vi "Get Tag.vi"(7 "IFDO":T4(c390), 8 "error in 2":errorcluster, 9 "byte order (0:big-endian, network order)":T1(ring), 10 "Tag ID":T2=254 items=["NewSubfileType"=254, "ImageWidth"=256, "ImageLength"=257, "BitsPerSample"=258, "Compression"=259, "PhotometricInterpretation"=262, "StripOffsets"=273, "SamplesPerPixel"=277, "RowsPerStrip"=278, "StripByteCounts"=279, "XResolution"=282, "YResolution"=283, "ResolutionUnit"=296, "ColorMap"=320, "PlanarrConfiguration"=284, "YCbCrCoefficients"=529, "YCbCrSubSampling"=530, "YCbCrPositioning"=531, "ReferenceBlackWhite"=532, "BadFaxLines"=326, "CleanFaxData"=327, "ConsecutiveBadFaxLines"=328], 11 "File Refnum":refnum<file>) -> (0 "error out":errorcluster, 1 "Tag found?":bool, 2 "Data":variant, 3 "refnum out":refnum<file>)   [LabVIEW 2020, in "LV Tiff.lvlib"]
uses:
  LV Tiff.lvlib
  Tiff Data Type.ctl
  Tiff Tags.ctl
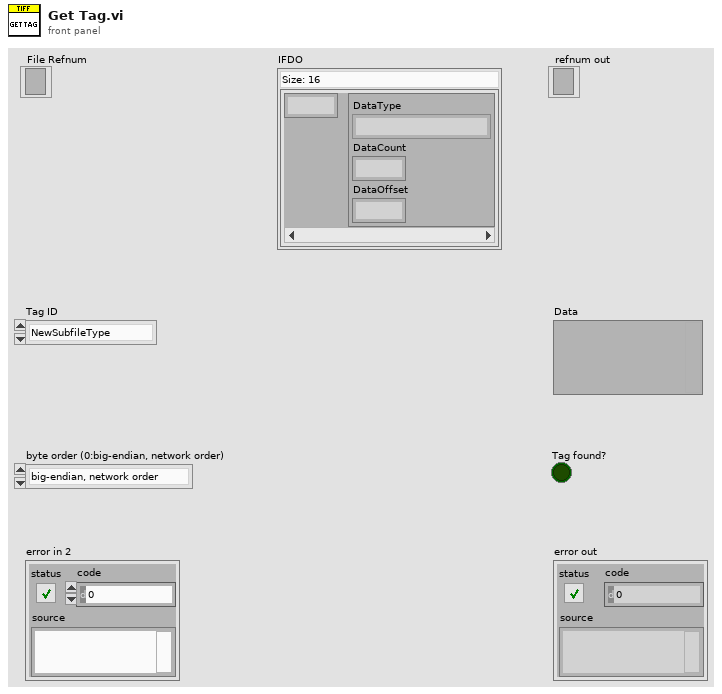
[diagram p1: front panel]
types:
  T1 = enum16{"big-endian, network order", "native, host order", "little-endian"}
  T2 = typedef "LV Tiff.lvlib/Tiff Tags.ctl" = u16
  T3 = typedef "LV Tiff.lvlib/Tiff Data Type.ctl" = enum16{"Null", "BYTE", "ASCII", "SHORT", "LONG", "RATIONAL", "SBYTE", "UNDEFINE", "SSHORT", "SLONG", "SRATIONAL", "FLOAT", "DOUBLE"}
  T4 = map{u16, cluster{"DataType":T3, "DataCount":u32, "DataOffset":u32}}
  T5 = map{u16, cluster{"string array[0]":string, T3[]}}
  T6 = cluster{"DataType":T3, "DataCount":u32, "DataOffset":u32}
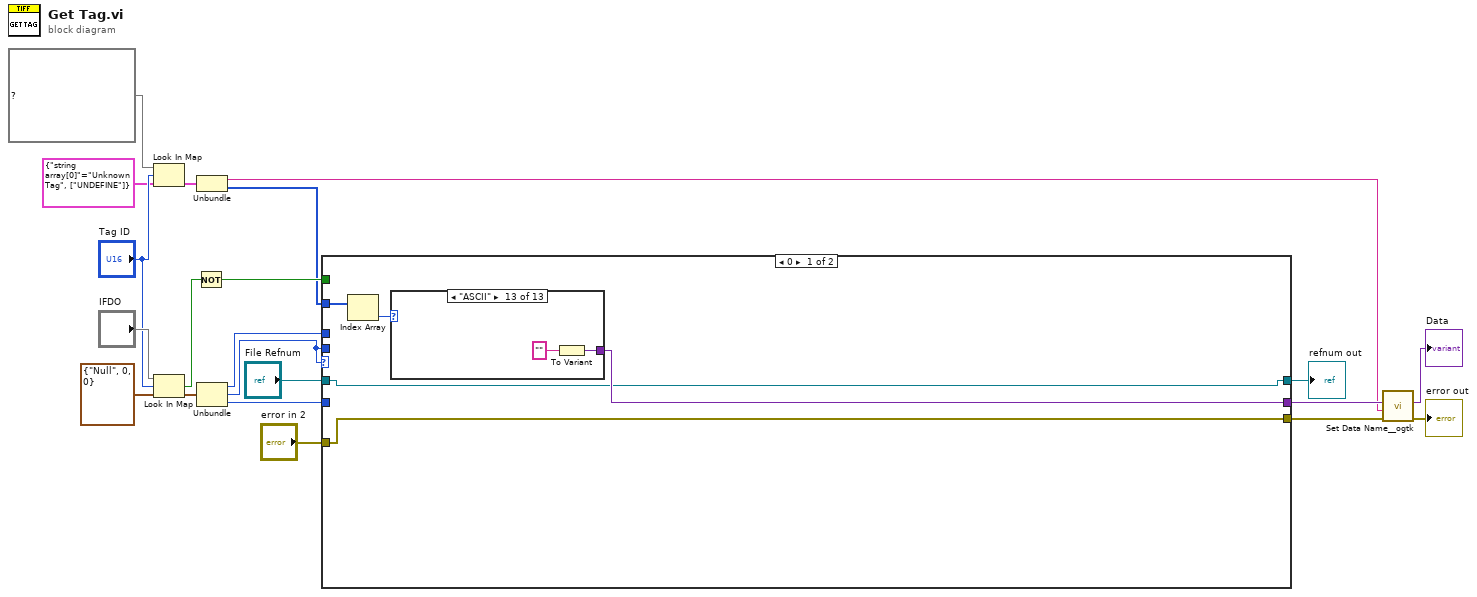
[diagram p0: block diagram]
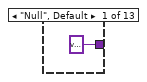
[diagram p2: hidden frame]
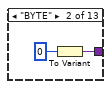
[diagram p3: hidden frame]
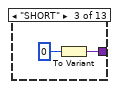
[diagram p4: hidden frame]
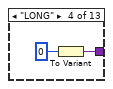
[diagram p5: hidden frame]
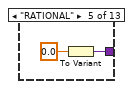
[diagram p6: hidden frame]
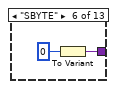
[diagram p7: hidden frame]
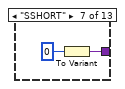
[diagram p8: hidden frame]
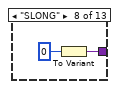
[diagram p9: hidden frame]
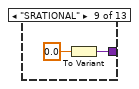
[diagram p10: hidden frame]
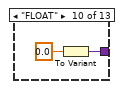
[diagram p11: hidden frame]
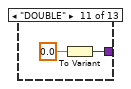
[diagram p12: hidden frame]
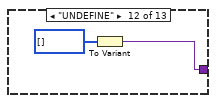
[diagram p13: hidden frame]
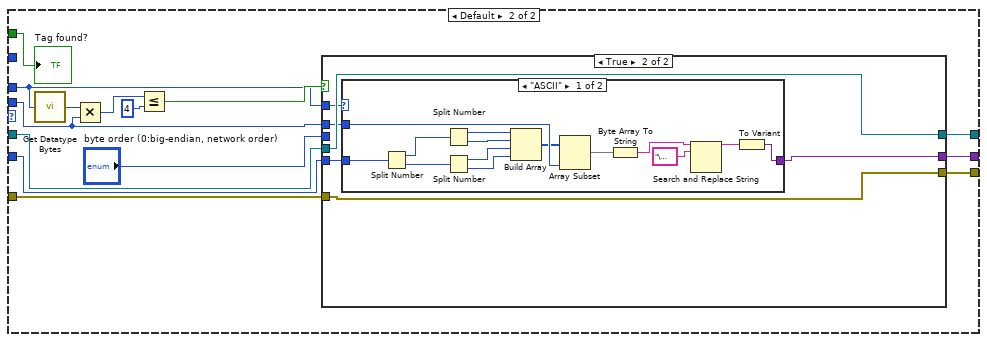
[diagram p14: hidden frame]
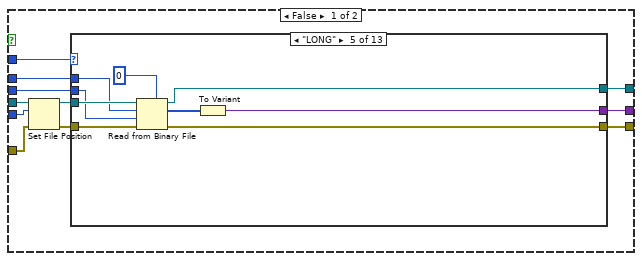
[diagram p15: hidden frame]
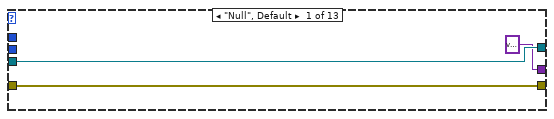
[diagram p16: hidden frame]
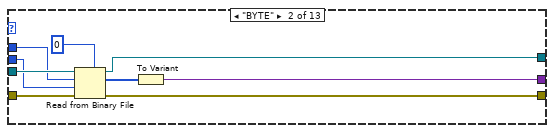
[diagram p17: hidden frame]
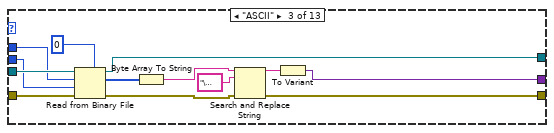
[diagram p18: hidden frame]
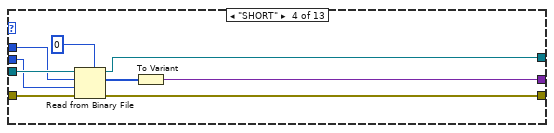
[diagram p19: hidden frame]
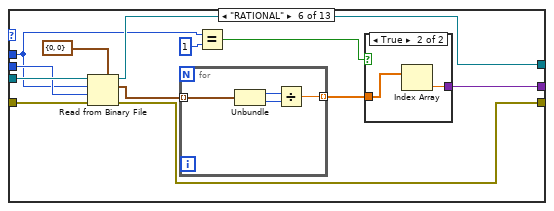
[diagram p20: hidden frame]
diagram:
  n1 = Look In Map(map=T5 {254={"string array[0]"="NewSubFileType", [enum."LONG"]}, 255={"string array[0]"="SubFileType", [enum."SHORT"]}, 256={"string array[0]"="ImageWidth", [enum."SHORT", enum."LONG"]}, 257={"string array[0]"="ImageHeight", [enum."SHORT", enum."LONG"]}, 258={"string array[0]"="BitsPerSample", [enum."SHORT"]}, 259={"string array[0]"="Compression", [enum."SHORT"]}, 262={"string array[0]"="PhotometricInterpretation", [enum."SHORT"]}, 263={"string array[0]"="Thresholding", [enum."SHORT"]}, 264={"string array[0]"="CellWidth", [enum."SHORT"]}, 265={"string array[0]"="CellLength", [enum."SHORT"]}, 266={"string array[0]"="FillOrder", [enum."SHORT"]}, 269={"string array[0]"="DocumentName", [enum."ASCII"]}, 270={"string array[0]"="ImageDescription", [enum."ASCII"]}, 271={"string array[0]"="Make", [enum."ASCII"]}, 272={"string array[0]"="Model", [enum."ASCII"]}, 273={"string array[0]"="StripOffsets", [enum."SHORT", enum."LONG"]}, 274={"string array[0]"="Orientation", [enum."SHORT"]}, 277={"string array[0]"="SamplesPerPixel", [enum."SHORT"]}, 278={"string array[0]"="RowsPerStrip", [enum."SHORT", enum."LONG"]}, 279={"string array[0]"="StripByteCounts", [enum."LONG", enum."SHORT"]}, 280={"string array[0]"="MinSampleValue", [enum."SHORT"]}, 281={"string array[0]"="MaxSampleValue", [enum."SHORT"]}, 282={"string array[0]"="XResolution", [enum."RATIONAL"]}, 283={"string array[0]"="YResolution", [enum."RATIONAL"]}, 284={"string array[0]"="PlanarConfiguration", [enum."SHORT"]}, 285={"string array[0]"="PageName", [enum."ASCII"]}, 286={"string array[0]"="XPosition", [enum."RATIONAL"]}, 287={"string array[0]"="YPosition", [enum."RATIONAL"]}, 288={"string array[0]"="FreeOffsets", [enum."LONG"]}, 289={"string array[0]"="FreeByteCounts", [enum."LONG"]}, 290={"string array[0]"="GrayResponseUnit", [enum."SHORT"]}, 291={"string array[0]"="GrayResponseCurve", [enum."SHORT"]}, 292={"string array[0]"="T4Options[2]", [enum."LONG"]}, 293={"string array[0]"="T6Options[3]", [enum."LONG"]}, 296={"string array[0]"="ResolutionUnit", [enum."SHORT"]}, 297={"string array[0]"="PageNumber", [enum."SHORT"]}, 300={"string array[0]"="ColorResponseUnit", [enum."SHORT"]}, 301={"string array[0]"="TransferFunction[4]", [enum."SHORT"]}, 305={"string array[0]"="Software", [enum."ASCII"]}, 306={"string array[0]"="DateTime", [enum."ASCII"]}, 315={"string array[0]"="Artist", [enum."ASCII"]}, 316={"string array[0]"="HostComputer", [enum."ASCII"]}, 317={"string array[0]"="Predictor", [enum."SHORT"]}, 318={"string array[0]"="WhitePoint", [enum."RATIONAL"]}, 319={"string array[0]"="PrimaryChromaticities", [enum."RATIONAL"]}, 320={"string array[0]"="ColorMap", [enum."SHORT"]}, 321={"string array[0]"="HalftoneHints", [enum."SHORT"]}, 322={"string array[0]"="TileWidth", [enum."SHORT", enum."LONG"]}, 323={"string array[0]"="TileLength", [enum."SHORT", enum."LONG"]}, 324={"string array[0]"="TileOffsets", [enum."LONG"]}, 325={"string array[0]"="TileByteCounts", [enum."SHORT", enum."LONG"]}, 326={"string array[0]"="BadFaxLines", [enum."SHORT", enum."LONG"]}, 327={"string array[0]"="CleanFaxData", [enum."SHORT"]}, 328={"string array[0]"="ConsecutiveBadFaxLines", [enum."LONG", enum."SHORT"]}, 332={"string array[0]"="InkSet", [enum."SHORT"]}, 333={"string array[0]"="InkNames", [enum."ASCII"]}, 334={"string array[0]"="NumberOfInks", [enum."SHORT"]}, 336={"string array[0]"="DotRange", [enum."BYTE", enum."SHORT"]}, 337={"string array[0]"="TargetPrinter", [enum."ASCII"]}, 338={"string array[0]"="ExtraSamples", [enum."BYTE"]}, 339={"string array[0]"="SampleFormat", [enum."SHORT"]}, 340={"string array[0]"="SMinSampleValue", [enum."Null"]}, 341={"string array[0]"="SMaxSampleValue", [enum."Null"]}, 342={"string array[0]"="TransferRange", [enum."SHORT"]}, 512={"string array[0]"="JPEGProc", [enum."SHORT"]}, 513={"string array[0]"="JPEGInterchangeFormat", [enum."LONG"]}, 514={"string array[0]"="JPEGInterchangeFormatLength", [enum."LONG"]}, 515={"string array[0]"="JPEGRestartInterval", [enum."SHORT"]}, 517={"string array[0]"="JPEGLosslessPredictors", [enum."SHORT"]}, 518={"string array[0]"="JPEGPointTransforms", [enum."SHORT"]}, 519={"string array[0]"="JPEGQTables", [enum."LONG"]}, 520={"string array[0]"="JPEGDCTTables", [enum."LONG"]}, 521={"string array[0]"="JPEGACTTables", [enum."LONG"]}, 529={"string array[0]"="YCbCrCoefficients", [enum."RATIONAL"]}, 530={"string array[0]"="YCbCrSubSampling", [enum."SHORT"]}, 531={"string array[0]"="YCbCrPositioning", [enum."SHORT"]}, 532={"string array[0]"="ReferenceBlackWhite", [enum."LONG"]}, 33432={"string array[0]"="Copyright", [enum."ASCII"]}} ("Map 2"), key="Tag ID", default value=cluster{"string array[0]":string, T3[]} {"string array[0]"="Unknown Tag", [enum."UNDEFINE"]}) -> (value=w9:cluster{"string array[0]":string, T3[]})  [unwired: 1 out]
  n2 = Look In Map(map="IFDO", key="Tag ID", default value=T6 {"DataType"=enum."Null", "DataCount"=0, "DataOffset"=0}) -> (key not found?=w16:bool, value=w20:T6)
  n3 = Not(x=w16) -> (.not. x?=w17:bool)
  n4 = Unbundle(w9) -> ("string array[0]"=w6:string, w3:T3[])
  n5 = Unbundle(w20) -> ("DataType"=w14:T3, "DataCount"=w4:u32, "DataOffset"=w15:u32)
  n6 = case shown="0" w4 {
    tunnel: [w23 w65] -> w19
    tunnel: [w22 w64] -> w18
    tunnel: w17 -> [_ w63]
    tunnel: w15 -> [_ w57]
    tunnel: w14 -> [_ w56]
    tunnel: w4 -> [_ w55]
    tunnel: [w24 w54] -> w11
    tunnel: w3 -> [w26 _]
    tunnel: "File Refnum" -> [w23 w53]
    tunnel: "error in 2" -> [w22 w52]
    frame 0 {
      n7 = Index Array(array=w26) -> (element=w25:T3)  [unwired: 1 in]
      n8 = case shown="\"ASCII\"" w25 {
        tunnel: [variant ("Variant") w28 w30 w32 w34 w36 w38 w40 w42 w44 w46 w48 w50] -> w24
        frame "Null", Default {
        }
        frame "BYTE" {
          n9 = To Variant(anything=u8 0) -> (Variant=w28:variant)
        }
        frame "SHORT" {
          n10 = To Variant(anything=u16 0) -> (Variant=w30:variant)
        }
        frame "LONG" {
          n11 = To Variant(anything=u32 0) -> (Variant=w32:variant)
        }
        frame "RATIONAL" {
          n12 = To Variant(anything=0.0) -> (Variant=w34:variant)
        }
        frame "SBYTE" {
          n13 = To Variant(anything=i8 0) -> (Variant=w36:variant)
        }
        frame "SSHORT" {
          n14 = To Variant(anything=i16 0) -> (Variant=w38:variant)
        }
        frame "SLONG" {
          n15 = To Variant(anything=0) -> (Variant=w40:variant)
        }
        frame "SRATIONAL" {
          n16 = To Variant(anything=0.0) -> (Variant=w42:variant)
        }
        frame "FLOAT" {
          n17 = To Variant(anything=sgl 0.0) -> (Variant=w44:variant)
        }
        frame "DOUBLE" {
          n18 = To Variant(anything=0.0) -> (Variant=w46:variant)
        }
        frame "UNDEFINE" {
          n19 = To Variant(anything=u8[] []) -> (Variant=w48:variant)
        }
        frame "ASCII" {
          n20 = To Variant(anything="") -> (Variant=w50:variant)
        }
      }
    }
    frame Default {
      n21 = call "Get Datatype Bytes.vi"("DataType"=w56) -> ("N Bytes"=w61:u8)
      n22 = Multiply(x=w61, y=w55) -> (x*y=w60:u32)
      n23 = Less Or Equal?(x=w60, y=u32 4) -> (x <= y?=w58:bool)
      n24 = case shown="True" w58 {
        tunnel: [w66 w215] -> w54
        tunnel: w57 -> [w70 w216]
        tunnel: w53 -> [w76 w220]
        tunnel: [w74 w220] -> w65
        tunnel: w52 -> [w73 w219]
        tunnel: [w71 w219] -> w64
        tunnel: w56 -> [w69 w217]
        tunnel: w55 -> [w68 w218]
        tunnel: "byte order (0:big-endian, network order)" -> [w67 _]
        frame False {
          n25 = Set File Position(offset (in bytes) (0)=w70, refnum=w76, error in=w73) -> (refnum out=w75:refnum<file>, error out=w72:errorcluster)  [unwired: 1 in]
          n26 = case shown="\"LONG\"" w69 {
            tunnel: w75 -> [w79 w88 w101 w110 w119 w131 w148 w157 w166 w175 w184 w193 w206]
            tunnel: [w79 w87 w100 w109 w118 w130 w147 w156 w165 w174 w183 w192 w205] -> w74
            tunnel: w72 -> [w77 w86 w99 w108 w117 w129 w146 w155 w164 w173 w182 w191 w204]
            tunnel: [w77 w85 w90 w107 w116 w128 w145 w154 w163 w172 w181 w190 w203] -> w71
            tunnel: w68 -> [_ w83 w97 w105 w114 w122 w144 w153 w162 w171 w180 w189 w196]
            tunnel: w67 -> [_ w82 w96 w104 w113 w127 w143 w152 w161 w170 w179 w188 w202]
            tunnel: [variant ("Variant") w80 w94 w103 w112 w126 w142 w151 w160 w169 w178 w187 w201] -> w66
            frame "Null", Default {
            }
            frame "BYTE" {
              n27 = Read from Binary File(5:u8 0, 8:w86, 9:w82, 10:w83, 11:w88) -> (0:w85:errorcluster, 2:w81:u8[], 3:w87:refnum<file>)  [unwired: 1 in, 1 out]
              n28 = To Variant(anything=w81) -> (Variant=w80:variant)
            }
            frame "ASCII" {
              n29 = Read from Binary File(5:u8 0, 8:w99, 9:w96, 10:w97, 11:w101) -> (0:w91:errorcluster, 2:w95:u8[], 3:w100:refnum<file>)  [unwired: 1 in, 1 out]
              n30 = Byte Array To String(unsigned byte array=w95) -> (string=w93:string)
              n31 = Search and Replace String(input string=w93, search string="\u0000", error in=w91) -> (result string=w92:string, error out=w90:errorcluster)  [unwired: 5 in, 2 out]
              n32 = To Variant(anything=w92) -> (Variant=w94:variant)
            }
            frame "SHORT" {
              n33 = Read from Binary File(5:u16 0, 8:w108, 9:w104, 10:w105, 11:w110) -> (0:w107:errorcluster, 2:w102:u16[], 3:w109:refnum<file>)  [unwired: 1 in, 1 out]
              n34 = To Variant(anything=w102) -> (Variant=w103:variant)
            }
            frame "LONG" {
              n35 = Read from Binary File(5:u32 0, 8:w117, 9:w113, 10:w114, 11:w119) -> (0:w116:errorcluster, 2:w111:u32[], 3:w118:refnum<file>)  [unwired: 1 in, 1 out]
              n36 = To Variant(anything=w111) -> (Variant=w112:variant)
            }
            frame "RATIONAL" {
              n37 = Read from Binary File(5:cluster{u32, u32} {0, 0}, 8:w129, 9:w127, 10:w122, 11:w131) -> (0:w128:errorcluster, 2:w124:cluster{u32, u32}[], 3:w130:refnum<file>)  [unwired: 1 in, 1 out]
              n38 = for {
                tunnel: w124 -> [w139] mode=indexing
                tunnel: [w136] -> w123 mode=indexing
                n39 = Unbundle(w139) -> (w138:u32, w137:u32)
                n40 = Divide(x=w138, y=w137) -> (x/y=w136:dbl)
              }
              n41 = Equal?(x=w122, y=u32 1) -> (x = y?=w120:bool)
              n42 = case shown="True" w120 {
                tunnel: [w133 w134] -> w126
                tunnel: w123 -> [w132 w135]
                frame False {
                  n43 = To Variant(anything=w132) -> (Variant=w133:variant)
                }
                frame True {
                  n44 = Index Array(array=w135) -> (element=w134:dbl)  [unwired: 1 in]
                }
              }
            }
            frame "SBYTE" {
              n45 = Read from Binary File(5:i8 0, 8:w146, 9:w143, 10:w144, 11:w148) -> (0:w145:errorcluster, 2:w141:i8[], 3:w147:refnum<file>)  [unwired: 1 in, 1 out]
              n46 = To Variant(anything=w141) -> (Variant=w142:variant)
            }
            frame "UNDEFINE" {
              n47 = Read from Binary File(5:u8 0, 8:w155, 9:w152, 10:w153, 11:w157) -> (0:w154:errorcluster, 2:w150:u8[], 3:w156:refnum<file>)  [unwired: 1 in, 1 out]
              n48 = To Variant(anything=w150) -> (Variant=w151:variant)
            }
            frame "SSHORT" {
              n49 = Read from Binary File(5:i16 0, 8:w164, 9:w161, 10:w162, 11:w166) -> (0:w163:errorcluster, 2:w159:i16[], 3:w165:refnum<file>)  [unwired: 1 in, 1 out]
              n50 = To Variant(anything=w159) -> (Variant=w160:variant)
            }
            frame "SLONG" {
              n51 = Read from Binary File(5:0, 8:w173, 9:w170, 10:w171, 11:w175) -> (0:w172:errorcluster, 2:w168:i32[], 3:w174:refnum<file>)  [unwired: 1 in, 1 out]
              n52 = To Variant(anything=w168) -> (Variant=w169:variant)
            }
            frame "FLOAT" {
              n53 = Read from Binary File(5:sgl 0.0, 8:w182, 9:w179, 10:w180, 11:w184) -> (0:w181:errorcluster, 2:w177:sgl[], 3:w183:refnum<file>)  [unwired: 1 in, 1 out]
              n54 = To Variant(anything=w177) -> (Variant=w178:variant)
            }
            frame "DOUBLE" {
              n55 = Read from Binary File(5:0.0, 8:w191, 9:w188, 10:w189, 11:w193) -> (0:w190:errorcluster, 2:w186:dbl[], 3:w192:refnum<file>)  [unwired: 1 in, 1 out]
              n56 = To Variant(anything=w186) -> (Variant=w187:variant)
            }
            frame "SRATIONAL" {
              n57 = Read from Binary File(5:cluster{i32, i32} {0, 0}, 8:w204, 9:w202, 10:w196, 11:w206) -> (0:w203:errorcluster, 2:w199:cluster{i32, i32}[], 3:w205:refnum<file>)  [unwired: 1 in, 1 out]
              n58 = for {
                tunnel: w199 -> [w214] mode=indexing
                tunnel: [w211] -> w198 mode=indexing
                n59 = Unbundle(w214) -> (w213:i32, w212:i32)
                n60 = Divide(x=w213, y=w212) -> (x/y=w211:dbl)
              }
              n61 = Equal?(x=w196, y=u32 1) -> (x = y?=w194:bool)
              n62 = case shown="True" w194 {
                tunnel: [w208 w209] -> w197
                tunnel: w198 -> [w207 w210]
                frame False {
                  n63 = To Variant(anything=w207) -> (Variant=w208:variant)
                }
                frame True {
                  n64 = Index Array(array=w210) -> (element=w209:dbl)  [unwired: 1 in]
                }
              }
              n65 = To Variant(anything=w197) -> (Variant=w201:variant)
            }
          }
        }
        frame True {
          n66 = case shown="\"ASCII\"" w217 {
            tunnel: w218 -> [w233 _]
            tunnel: w216 -> [w234 w236]
            tunnel: [w232 w235] -> w215
            frame "ASCII" {
              n67 = Split Number(x=w234) -> (hi(x)=w231:u16, lo(x)=w230:u16)
              n68 = Split Number(x=w231) -> (hi(x)=w229:u8, lo(x)=w228:u8)
              n69 = Split Number(x=w230) -> (hi(x)=w227:u8, lo(x)=w226:u8)
              n70 = Build Array(w229, w228, w227, w226) -> (w225:u8[])
              n71 = Array Subset(array=w225, length=w233) -> (w224:u8[])  [unwired: 1 in]
              n72 = Byte Array To String(unsigned byte array=w224) -> (string=w223:string)
              n73 = Search and Replace String(input string=w223, search string="\u0000") -> (result string=w222:string)  [unwired: 6 in, 3 out]
              n74 = To Variant(anything=w222) -> (Variant=w232:variant)
            }
            frame Default {
              n75 = To Variant(anything=w236) -> (Variant=w235:variant)
            }
          }
        }
      }
      "Tag found?" <- w63
    }
  }
  "refnum out" <- w19
  n76 = call <userlib>:"Set Data Name__ogtk.vi"("error in (no error)"=w18, "Data Name"=w6, "Data"=w11) -> ("error out"=→"error out":errorcluster, "Renamed Data"=→"Data":variant)  [unwired: 7 in]
